vi "Configure Operation Mode Core.vi"(8 "error in (no error)":errorcluster, 9 "operation mode (Continuous)":i32(ring) items=["Continuous", "Burst"], 10 "channel name (\"CHANNEL1\")":string="CHANNEL1", 11 "IVI_Fgen in":refnum<class "IVI_Fgen.lvclass">) -> (0 "error out":errorcluster, 3 "IVI_Fgen out":refnum<class "IVI_Fgen.lvclass">)   [LabVIEW 2015, in "IVI_Fgen.lvlib" / "IVI_Fgen.lvclass"]
doc: "This VI configures the operation mode of the function generator. The operation mode determines how the function generator produces output on a channel. For example, you can select to generate output continuously or to generate a discrete number of waveform cycles based on a trigger event."
uses:
  IVI_Fgen.lvclass
  IVI_Fgen.lvclass/IVI_Fgen.ctl
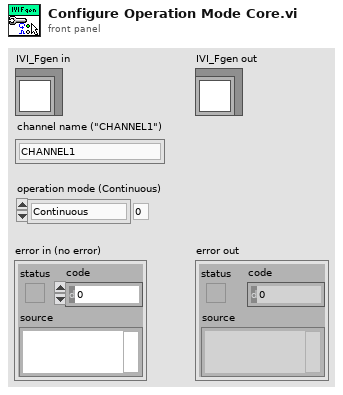
[diagram p1: front panel]
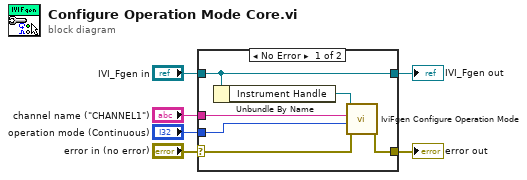
[diagram p0: block diagram]
diagram:
  n1 = case shown="No Error" "error in (no error)" {
    selector: "error in (no error)" -> [w10 w14]
    tunnel: [w9 w14] -> w5
    tunnel: [w12 w13] -> w3
    tunnel: "IVI_Fgen in" -> [w12 w13]
    tunnel: "channel name (\"CHANNEL1\")" -> [w8 _]
    tunnel: "operation mode (Continuous)" -> [w7 _]
    frame No Error {
      n2 = Unbundle By Name(w12) -> ("Instrument Handle"=w11:refnum<k15>)
      n3 = call <vilib>:"IviFgen Configure Operation Mode.vi"("error in (no error)"=w10, "operation mode (Continuous)"=w7, "channel name (\"CHANNEL1\")"=w8, "instrument handle"=w11) -> ("error out"=w9:errorcluster)  [unwired: 6 in, 1 out]
    }
    frame Error {
    }
  }
  "error out" <- w5
  "IVI_Fgen out" <- w3
